vi "RotationScaling.vi"(7 "InDeadband":bool, 10 "powerScale":dbl, 11 "Input":dbl) -> (3 "Output":dbl)   [LabVIEW 2020]
panel:
  in  "minimum":dbl=0.2
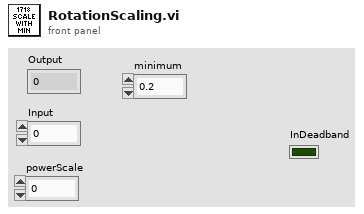
[diagram p1: front panel]
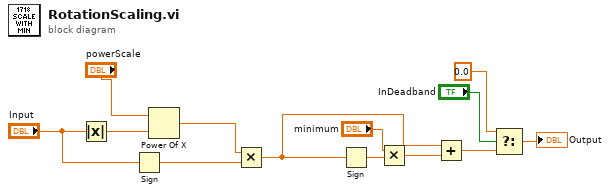
[diagram p0: block diagram]
diagram:
  n1 = Absolute Value(x="Input") -> (abs(x)=w11:dbl)
  n2 = Sign(1:"Input") -> (0:w10:dbl)
  n3 = Power Of X(1:w11, 2:"powerScale") -> (0:w9:dbl)
  n4 = Multiply(x=w9, y=w10) -> (x*y=w1:dbl)
  n5 = Sign(1:w1) -> (0:w5:dbl)
  n6 = Multiply(x="minimum", y=w5) -> (x*y=w6:dbl)
  n7 = Add(x=w1, y=w6) -> (x+y=w7:dbl)
  n8 = Select(t=0.0, s="InDeadband", f=w7) -> (s? t:f=→"Output":dbl)
